vi "FT10_Connect Unitherm Handler.vi"(8 "error in (no error)":errorcluster, 9 "Message Data":variant, 11 "Message Handling Cluster in":T1) -> (0 "error out":errorcluster, 2 "Unitherm Connected?":bool, 3 "Message Handling Cluster out":T1)   [LabVIEW 2024]
doc: "Opens or closes VISA connection to Unitherm."
uses:
  Controls/Control_Message Handling Cluster.ctl
  Controls/Control_M4X Connection.ctl
  Controls/Control_PXI-7854R FPGA Reference.ctl
  Controls/Control_Unitherm Connect Disconnect Cluster.ctl
  Controls/Control_Unitherm Connect Disconnect Bool.ctl
  Controls/Control_Unitherm VISA Resource.ctl
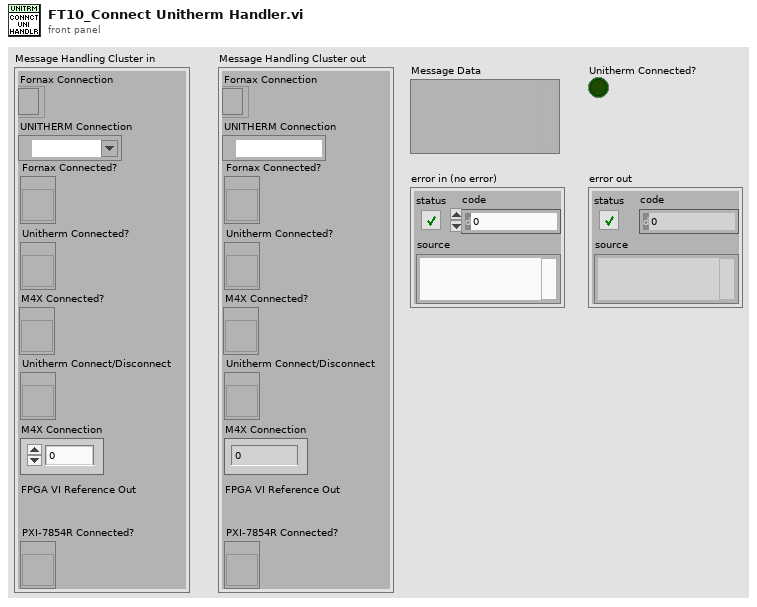
[diagram p1: front panel]
types:
  T1 = typedef "Control_Message Handling Cluster.ctl" = cluster{"Fornax Connection":refnum<k5>, "UNITHERM Connection":refnum<visa-resource-name>, "Fornax Connected?":refnum<vi>, "Unitherm Connected?":refnum<vi>, "M4X Connected?":refnum<vi>, "Unitherm Connect/Disconnect":refnum<vi>, "M4X Connection":T2, "PXI-7854R FPGA Reference":T3, "PXI-7854R Connected?":refnum<vi>}
  T2 = typedef "Control_M4X Connection.ctl" = u32
  T3 = typedef "Control_PXI-7854R FPGA Reference.ctl" = refnum<k20>
  T4 = typedef "Control_Unitherm Connect Disconnect Cluster.ctl" = cluster{"Unitherm Connect/Disconnect":T5, "Unitherm Refnum in":T6}
  T5 = typedef "Control_Unitherm Connect Disconnect Bool.ctl" = bool
  T6 = typedef "Control_Unitherm VISA Resource.ctl" = refnum<visa-resource-name>
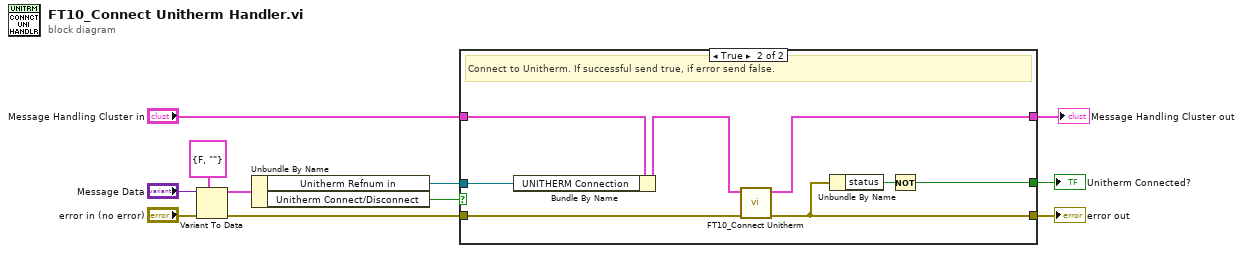
[diagram p0: block diagram]
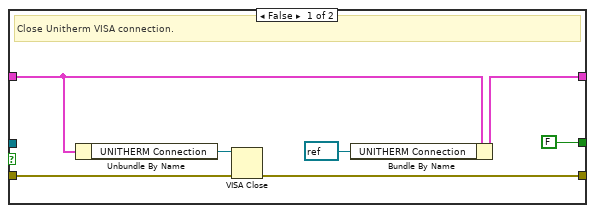
[diagram p2: hidden frame]
diagram:
  n1 = Variant To Data(error in="error in (no error)", type=T4 {"Unitherm Connect/Disconnect"=FALSE, "Unitherm Refnum in"=""}, Variant="Message Data") -> (data=w10:T4, error out=w9:errorcluster)
  n2 = Unbundle By Name(w10) -> ("Unitherm Refnum in"=w1:T6, "Unitherm Connect/Disconnect"=w2:T5)
  n3 = case shown="True" w2 {
    tunnel: [w14 w23] -> w5
    tunnel: [w17 w21] -> w6
    tunnel: "Message Handling Cluster in" -> [w18 w22]
    tunnel: w9 -> [w15 w24]
    tunnel: [FALSE w25] -> w11
    tunnel: w1 -> [_ w19]
    frame False {
      # "Close Unitherm VISA connection."
      n4 = Unbundle By Name(w18) -> ("UNITHERM Connection"=w13:refnum<visa-resource-name>)
      n5 = VISA Close(VISA resource name=w13, error in (no error)=w15) -> (error out=w14:errorcluster)
      n6 = Bundle By Name(cluster=w18, "UNITHERM Connection"=refnum<visa-resource-name> refnum) -> (w17:T1)
    }
    frame True {
      # "Connect to Unitherm. If successful send true, if error send false."
      n7 = Bundle By Name(cluster=w22, "UNITHERM Connection"=w19) -> (w20:T1)
      n8 = call "FT10_Connect Unitherm.vi"("error in (no error)"=w24, "Message Handling Cluster in"=w20) -> ("error out"=w23:errorcluster, "Message Handling Cluster out"=w21:T1)  [unwired: 8 in]
      n9 = Unbundle By Name(w23) -> ("status"=w26:bool)
      n10 = Not(x=w26) -> (.not. x?=w25:bool)
    }
  }
  "error out" <- w5
  "Message Handling Cluster out" <- w6
  "Unitherm Connected?" <- w11
